vi "Read Weekly Recur on_.vi"(8 "error in (no error)":errorcluster, 11 "Weekly in":refnum<class "Weekly.lvclass">) -> (0 "error out":errorcluster, 2 "Weekly Recur on:":T1 caption="Recur on:", 3 "Weekly out":refnum<class "Weekly.lvclass">)   [LabVIEW 2020]
uses:
  Weekly.lvclass/Weekly.ctl
  Weekly.lvclass
  C:/projects/budget_LabVIEW/Main Codeline/Software/Code/shared/ARecurrence/ARecurrence.lvclass
  C:/projects/budget_LabVIEW/Main Codeline/Software/Code/shared/IRecurrable/IRecurrable.lvclass
  C:/projects/budget_LabVIEW/Main Codeline/Software/Code/shared/Weekly/Weekly.lvclass
  Weekly Recurrence Type STYP.ctl
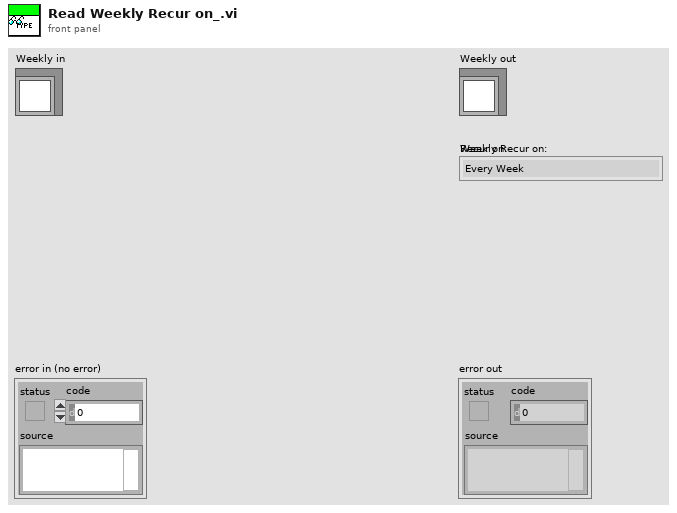
[diagram p1: front panel]
types:
  T1 = typedef "Weekly.lvclass/Weekly Recurrence Type STYP.ctl" = enum16{"Every Week", "Only Specific Weeks of a Month"}
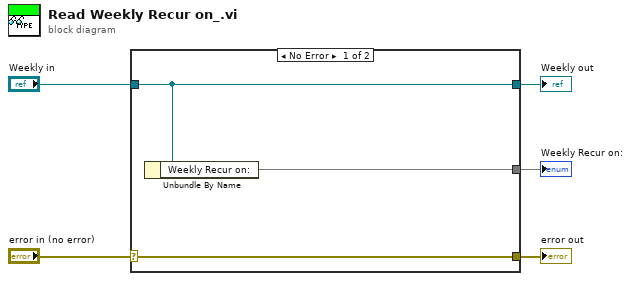
[diagram p0: block diagram]
diagram:
  n1 = case shown="No Error" "error in (no error)" {
    selector: "error in (no error)" -> [w8 w9]
    tunnel: [w8 w9] -> w4
    tunnel: [w7 w10] -> w2
    tunnel: "Weekly in" -> [w7 w10]
    tunnel: [w6 _] -> w1
    frame No Error {
      n2 = Unbundle By Name(w7) -> ("Weekly Recur on:"=w6)
    }
    frame Error {
    }
  }
  "error out" <- w4
  "Weekly out" <- w2
  "Weekly Recur on:" <- w1
